vi "ReadWriteTopicData.vi"(3 "error in (no error)":errorcluster, 4 "timeout ms (1000)":i32=1000, 5 "connection ID in":refnum<k5>) -> (0 "error out":errorcluster, 1 "data out":string, 2 "connection ID out":refnum<k5>)   [LabVIEW 2013]
uses:
  parsing/primitives/subs/parse_u32_scalar.vi
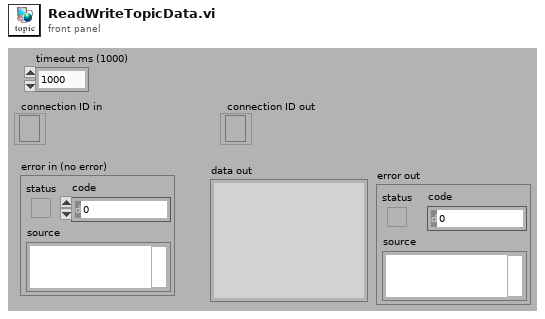
[diagram p1: front panel]
types:
  T1 = enum16{"Standard", "Buffered", "CRLF", "Immediate"}
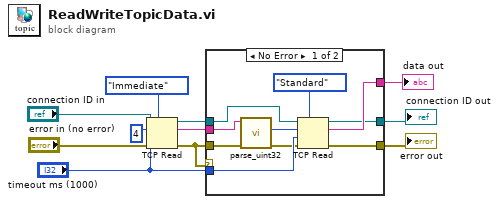
[diagram p0: block diagram]
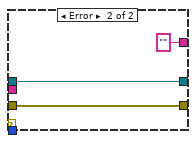
[diagram p2: hidden frame]
diagram:
  n1 = TCP Read(connection ID="connection ID in", bytes to read=4, error in (no error)="error in (no error)", 7:T1."Immediate" ("mode (standard)"), 9:"timeout ms (1000)") -> (connection ID out=w6:refnum<k5>, data out=w3:string, error out=w2:errorcluster)
  n2 = case shown="No Error" w2 {
    tunnel: [w21 "" ("data out")] -> w11
    tunnel: [w20 w23] -> w10
    tunnel: [w19 w24] -> w9
    tunnel: w2 -> [w14 w23]
    tunnel: w6 -> [w18 w24]
    tunnel: w3 -> [w12 _]
    tunnel: "timeout ms (1000)" -> [w16 _]
    frame No Error {
      n3 = call-poly "parse_uint32.vi"("error in"=w14, "msg in"=w12) -> ("error out"=w13:errorcluster, "number"=w15:u32)  [unwired: 3 in, 1 out]
      n4 = TCP Read(connection ID=w18, bytes to read=w15, error in (no error)=w13, 7:T1."Standard" ("mode (standard)"), 9:w16) -> (connection ID out=w19:refnum<k5>, data out=w21:string, error out=w20:errorcluster)
    }
    frame Error {
    }
  }
  "data out" <- w11
  "error out" <- w10
  "connection ID out" <- w9
